vi "myRIO_BRig_Host_v0,30.vi"() -> ()   [LabVIEW 2014]
panel:
  out "element":u16
  out "error_LoadPrevSettings":errorcluster caption="error out"
  in  "LoadPrevSettings":bool
  out "RunTime_seconds":u16
  out "RunTime_minutes":u16
  out "BlockL_T2R_cur":u16 caption="Trials2Reward"
  out "BlockL_BTPR_cur":u16 caption="BadTrialsPostReward"
  out "BlockL_T2R_avg":dbl caption="Trials2Reward" format="%#_3g"
  out "BlockL_BTPR_avg":dbl caption="BadTrialsPostReward" format="%#_3g"
  out "BlockR_T2R_cur":u16 caption="Trials2Reward"
  out "BlockR_BTPR_cur":u16 caption="BadTrialsPostReward"
  out "BlockR_T2R_avg":dbl caption="Trials2Reward" format="%#_3g"
  out "BlockR_BTPR_avg":dbl caption="BadTrialsPostReward" format="%#_3g"
  out "graph_ai1":dbl(graph)
  out "graph_ai0":dbl(graph)
  in  "dataIn_maxTrialsDisplayed":i32 caption="Number of Trials Displayed\n( 0 = all trials )"
  out "error_TCP":errorcluster
  in  "stop":bool
  in  "colorIn_timeout":u32(colorbox)=7468543 caption="Choice Timeout"
  in  "colorIn_wrong/cue":u32(colorbox)=16728618 caption="Wrong Choice or\nLicked During Cue"
  in  "colorIn_reward":u32(colorbox)=5898088 caption="Reward"
  in  "colorIn_unknown":u32(colorbox)=16449331 caption="Unknown Trial Status"
  out "dataOut_plot":cluster{i32[], i32[]}[](graph)
  out "iTrial":i32
  out "iBlock":i32
  # "Exp Stats"
  # "Current Block Stats"
  # "Trials 2 Reward\n\nBad Trials\nPost Reward"
  # "Left Spout    Right Spout"
  # "Run Time\n\n   minutes    seconds"
  # "Average Block Stats"
  # "Trials 2 Reward\n\nBad Trials\nPost Reward"
  # "Left Spout    Right Spout"
  # "If you get ERROR 5 related to opening a file, press CONTINUE"
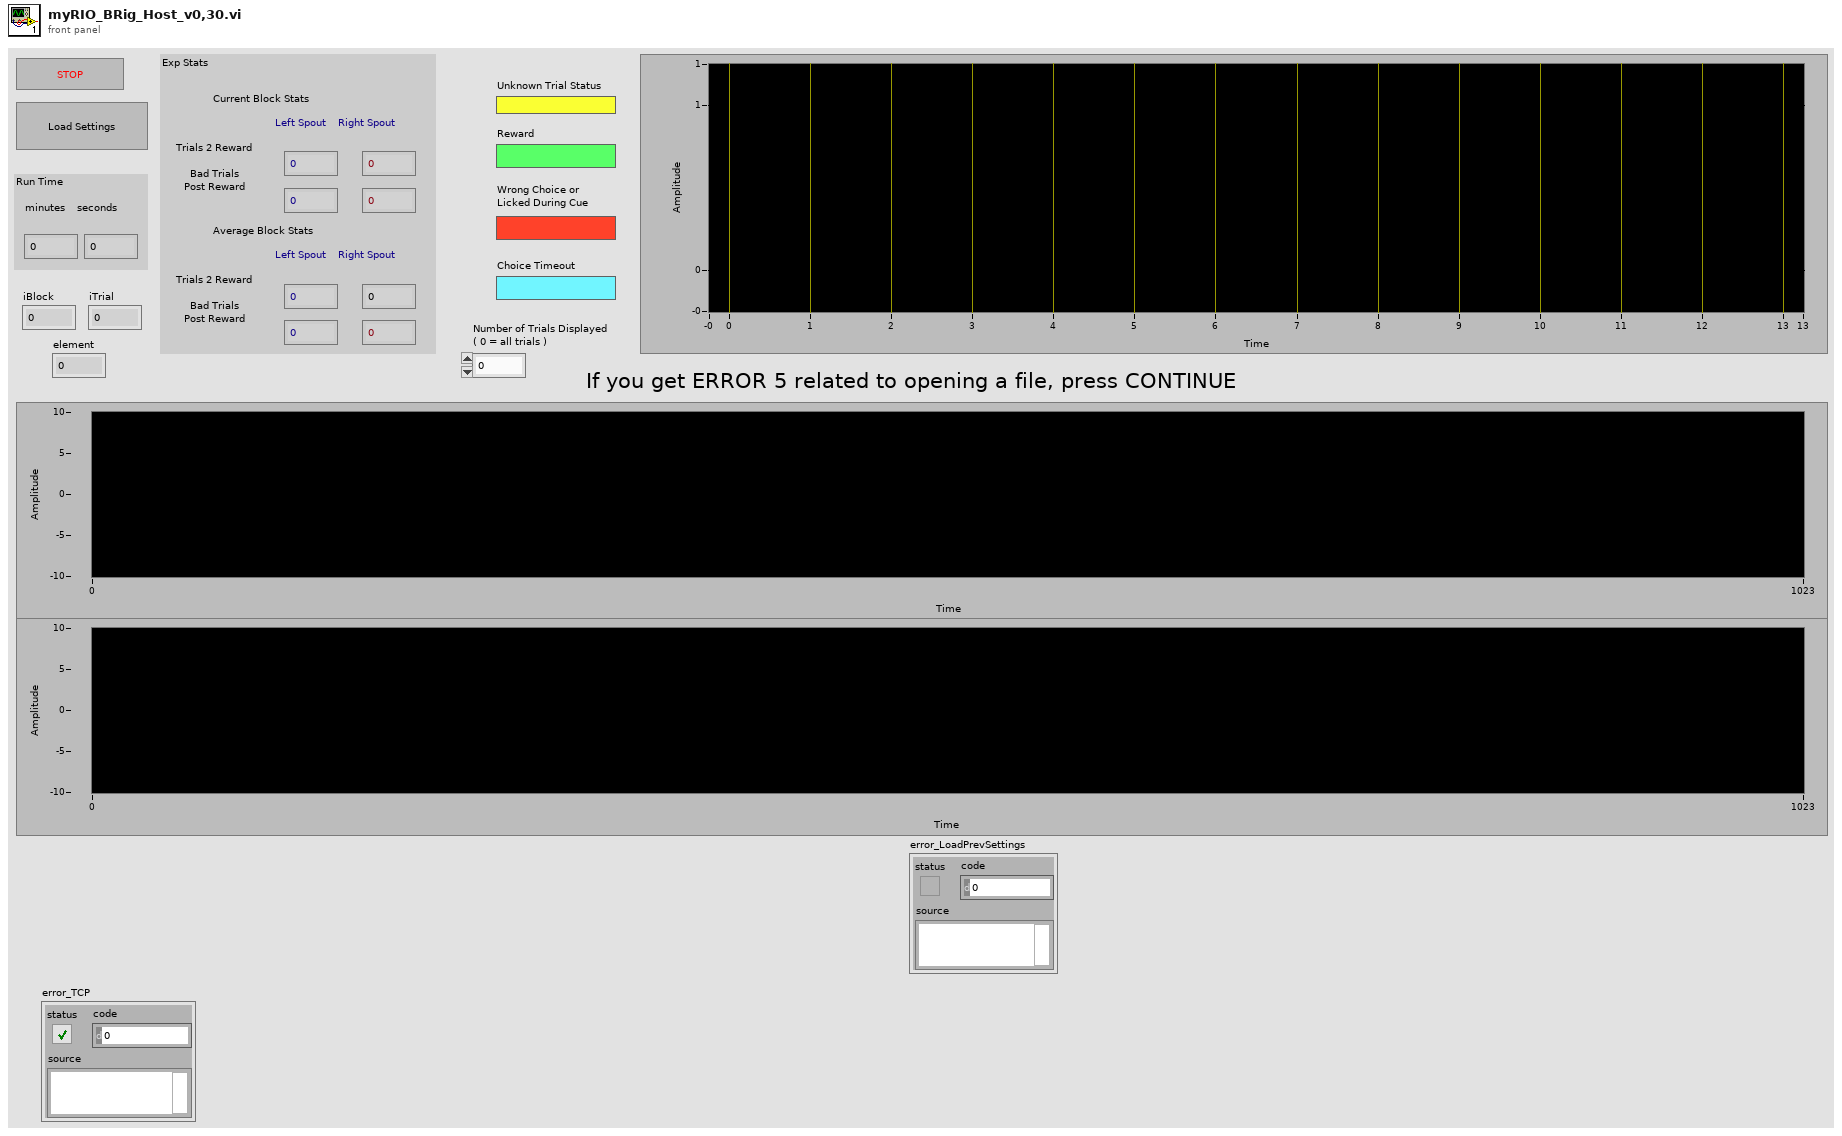
[diagram p1: front panel]
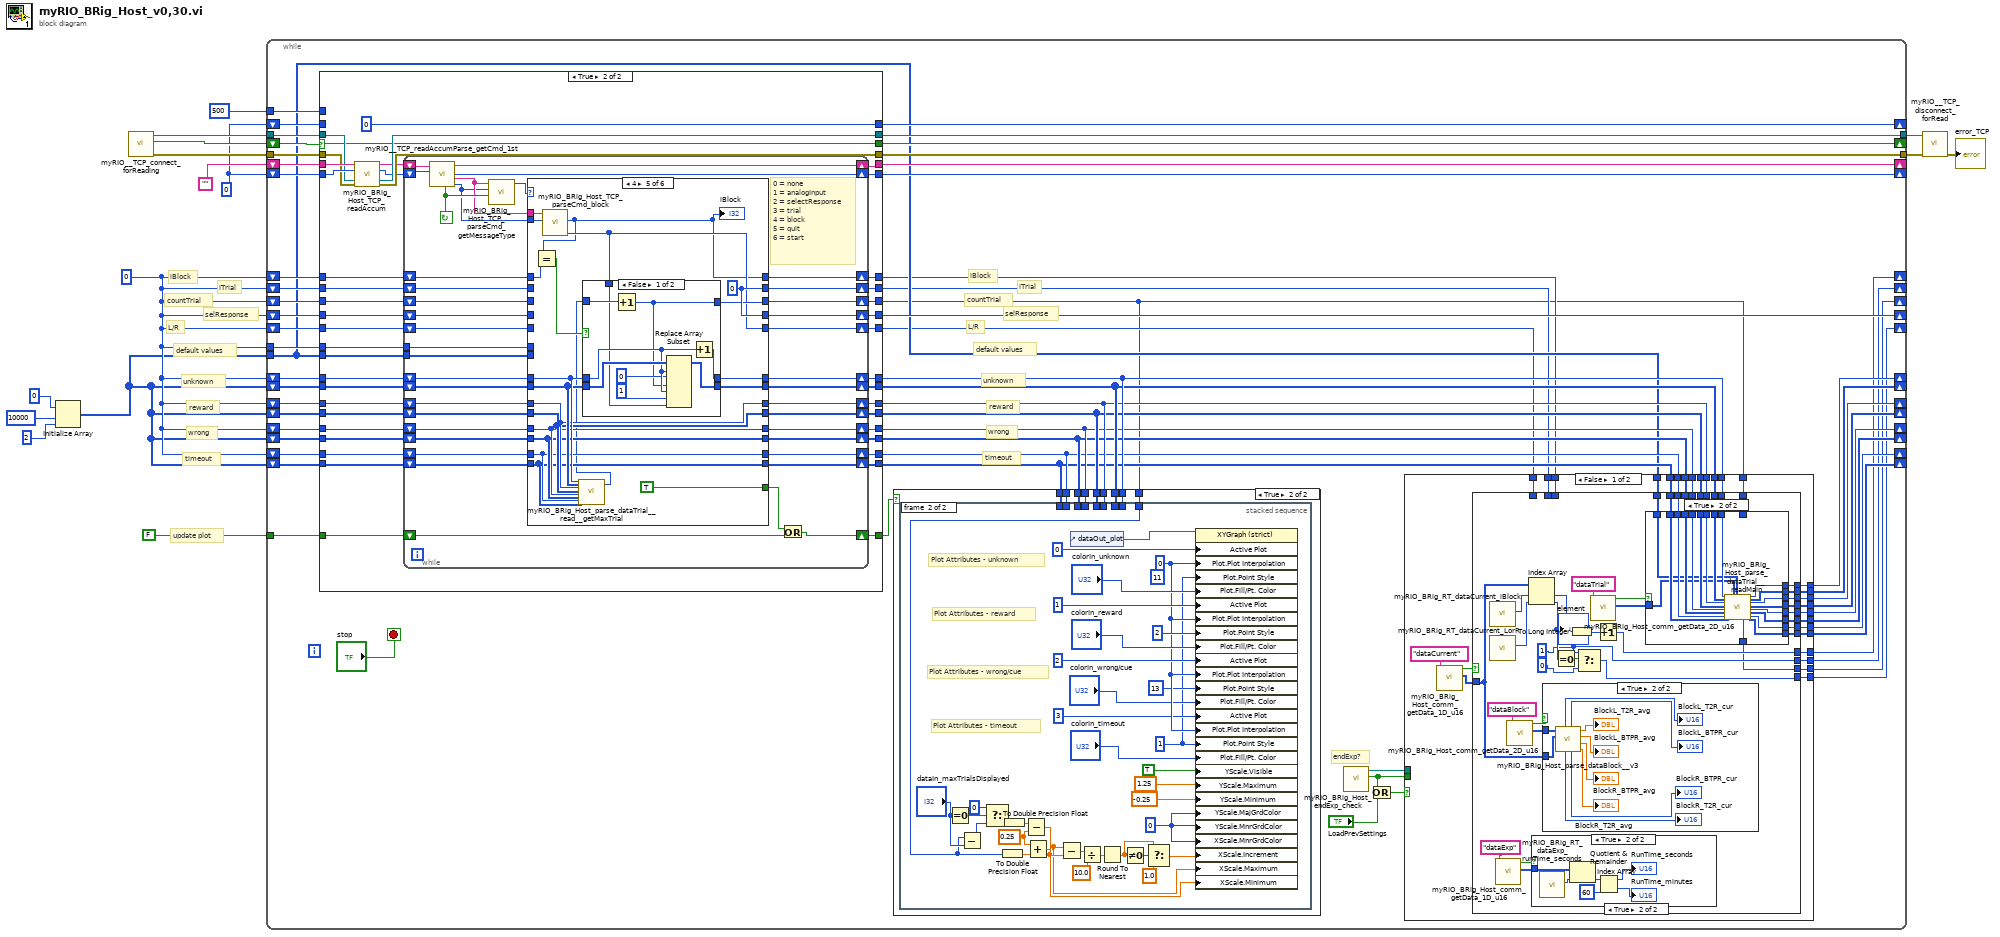
[diagram p0: block diagram]
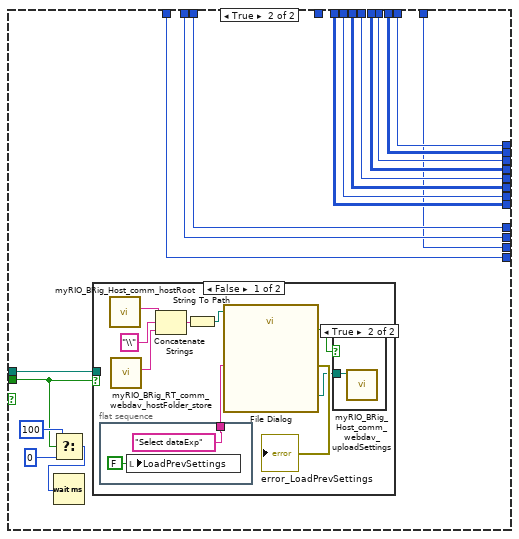
[diagram p6: hidden frame]
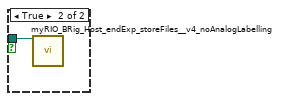
[diagram p8: hidden frame]
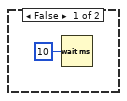
[diagram p9: hidden frame]
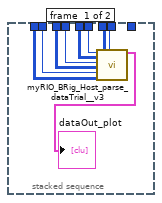
[diagram p10: hidden frame]
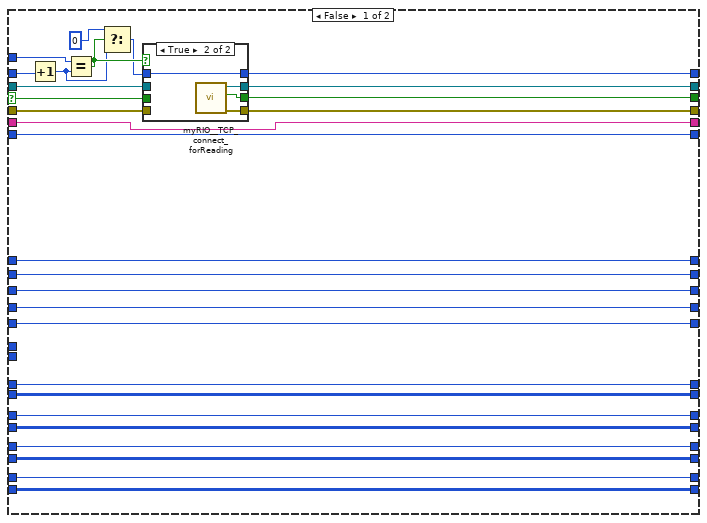
[diagram p11: hidden frame]
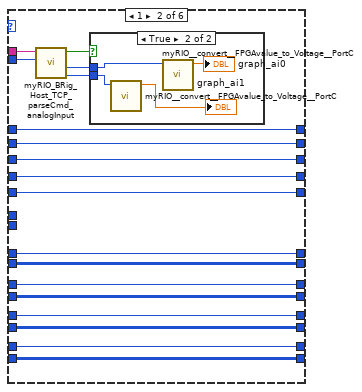
[diagram p14: hidden frame]
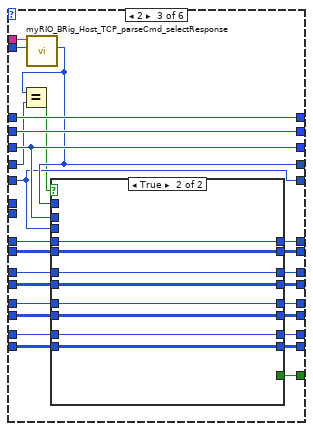
[diagram p16: hidden frame]
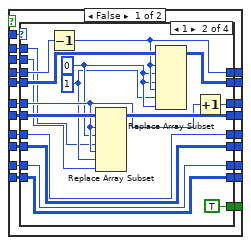
[diagram p17: hidden frame]
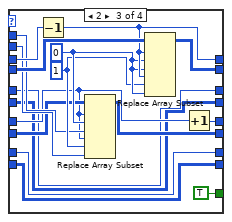
[diagram p19: hidden frame]
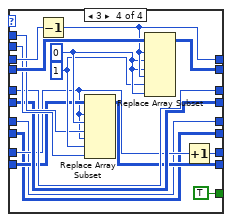
[diagram p20: hidden frame]
diagram:
  w2 = 0
  w11 = 0
  # "default values"
  # "update plot"
  # "timeout"
  # "wrong"
  # "reward"
  # "unknown"
  # "L/R"
  # "selResponse"
  # "countTrial"
  # "iBlock"
  # "iTrial"
  n1 = Initialize Array(0 ("element"), 10000 ("dimension size"), 2 ("dimension size")) -> (w1:i32[][])
  n2 = call "myRIO__TCP_connect_forReading.vi"() -> ("output_error"=w13:errorcluster, "output_connected"=w14:bool, "output_hTCP"=w15:refnum<k5>)  [unwired: 9 in]
  n3 = while {
    tunnel: w15 -> [w74]
    tunnel: w13 -> [w72]
    shift-right: [w65] -> _
    shift-left: w11 -> [w70]
    shift-right: [w66] -> _
    shift-left: "" -> [w71]
    shift-right: [w67] -> _
    shift-left: w14 -> [w73]
    shift-right: [w68] -> _
    shift-left: w11 -> [w75]
    tunnel: 500 ("y") -> [w69]
    shift-right: [w18] -> _
    shift-left: w2 -> [w64]
    shift-right: [w19] -> _
    shift-left: w2 -> [w63]
    shift-right: [w16] -> _
    shift-left: w2 -> [w62]
    shift-right: [w50] -> _
    shift-left: w2 -> [w61]
    shift-right: [w23] -> _
    shift-left: w2 -> [w60]
    shift-right: [w31] -> _
    shift-left: w2 -> [w59]
    shift-right: [w30] -> _
    shift-left: w1 -> [w58]
    shift-right: [w29] -> _
    shift-left: w2 -> [w57]
    shift-right: [w28] -> _
    shift-left: w1 -> [w56]
    shift-right: [w27] -> _
    shift-left: w2 -> [w55]
    shift-right: [w26] -> _
    shift-left: w1 -> [w54]
    shift-right: [w25] -> _
    shift-left: w2 -> [w53]
    shift-right: [w24] -> _
    shift-left: w1 -> [w52]
    tunnel: [w48] -> w5
    tunnel: [w47] -> w4
    tunnel: FALSE -> [w51]
    tunnel: w2 -> [w45]
    tunnel: w1 -> [w32]
    stop <- "stop" stop-if-true
    # "default values"
    # "timeout"
    # "wrong"
    # "reward"
    # "unknown"
    # "L/R"
    # "selResponse"
    # "countTrial"
    # "iBlock"
    # "iTrial"
    # "endExp?"
    n4 = case shown="True" w73 {
      selector: w73 -> [w305 w354]
      tunnel: w71 -> [w299 w360]
      tunnel: w70 -> [w300 w359]
      tunnel: [w299 w350] -> w66
      tunnel: [w300 w349] -> w65
      tunnel: w74 -> [w306 w358]
      tunnel: [w309 w357] -> w48
      tunnel: w72 -> [w304 w356]
      tunnel: [w308 w355] -> w47
      tunnel: [w307 w354] -> w67
      tunnel: w75 -> [w310 _]
      tunnel: [w298 0] -> w68
      tunnel: w69 -> [w297 _]
      tunnel: w64 -> [w296 w348]
      tunnel: w63 -> [w295 w347]
      tunnel: w62 -> [w294 w346]
      tunnel: w61 -> [w293 w345]
      tunnel: w60 -> [w292 w344]
      tunnel: w59 -> [w291 w343]
      tunnel: w58 -> [w290 w342]
      tunnel: w57 -> [w289 w341]
      tunnel: w56 -> [w288 w340]
      tunnel: w55 -> [w287 w339]
      tunnel: w54 -> [w286 w338]
      tunnel: w53 -> [w285 w337]
      tunnel: w52 -> [w284 w336]
      tunnel: w51 -> [_ w335]
      tunnel: [_ w334] -> w49
      tunnel: [w296 w333] -> w22
      tunnel: [w295 w332] -> w21
      tunnel: [w294 w331] -> w17
      tunnel: [w293 w330] -> w50
      tunnel: [w292 w329] -> w20
      tunnel: [w291 w328] -> w40
      tunnel: [w290 w327] -> w39
      tunnel: [w289 w326] -> w38
      tunnel: [w288 w325] -> w37
      tunnel: [w287 w324] -> w36
      tunnel: [w286 w323] -> w35
      tunnel: [w285 w322] -> w34
      tunnel: [w284 w321] -> w33
      tunnel: w45 -> [_ w320]
      tunnel: w32 -> [_ w319]
      frame False {
        n5 = Increment(x=w310) -> (x+1=w283:i32)
        n6 = Equal?(x=w297, y=w283) -> (x = y?=w303:bool)
        n7 = Select(t=0, s=w303, f=w283) -> (s? t:f=w301:i32)
        n8 = case shown="True" w303 {
          tunnel: w301 -> [w311 w315]
          tunnel: [w314 w318] -> w309
          tunnel: [w312 w317] -> w308
          tunnel: [w313 w316] -> w307
          tunnel: w306 -> [w314 _]
          tunnel: w305 -> [w313 _]
          tunnel: w304 -> [w312 _]
          tunnel: [w311 w315] -> w298
          frame False {
          }
          frame True {
            n9 = call "myRIO__TCP_connect_forReading.vi"() -> ("output_error"=w317:errorcluster, "output_connected"=w316:bool, "output_hTCP"=w318:refnum<k5>)  [unwired: 9 in]
          }
        }
      }
      frame True {
        n10 = call "myRIO_BRig_Host_TCP_readAccum.vi"("input_strAccum"=w360, "input_count"=w359, "input_handle_TCP"=w358, "input_error"=w356) -> ("output_strAccum"=w352:string, "output_count"=w351:i32, "output_handle_TCP"=w357:refnum<k5>, "output_error"=w355:errorcluster)  [unwired: 8 in]
        n11 = while {
          shift-right: [w397] -> w350
          shift-left: w352 -> [w399]
          shift-right: [w396] -> w349
          shift-left: w351 -> [w398]
          shift-right: [w388] -> w333
          shift-left: w348 -> [w391]
          shift-right: [w387] -> w332
          shift-left: w347 -> [w390]
          shift-right: [w386] -> w331
          shift-left: w346 -> [w389]
          shift-right: [w384] -> w330
          shift-left: w345 -> [w385]
          shift-right: [w382] -> w329
          shift-left: w344 -> [w383]
          shift-right: [w380] -> w328
          shift-left: w343 -> [w381]
          shift-right: [w378] -> w327
          shift-left: w342 -> [w379]
          shift-right: [w371] -> w326
          shift-left: w341 -> [w377]
          shift-right: [w370] -> w325
          shift-left: w340 -> [w376]
          shift-right: [w369] -> w324
          shift-left: w339 -> [w375]
          shift-right: [w368] -> w323
          shift-left: w338 -> [w374]
          shift-right: [w366] -> w321
          shift-left: w336 -> [w372]
          shift-right: [w367] -> w322
          shift-left: w337 -> [w373]
          shift-right: [w363] -> w334
          shift-left: w335 -> [w365]
          tunnel: w320 -> [w362]
          tunnel: w319 -> [w361]
          stop <- w395 continue-if-true
          # "0 = none\n1 = analogInput\n2 = selectResponse\n3 = trial\n4 = block\n5 = quit\n6 = start"
          n12 = call "myRIO__TCP_readAccumParse_getCmd_1st.vi"("input_count"=w398, "input_strAccum"=w399) -> ("output_countCmd"=w393:i32, "output_strCmd"=w394:string, "output_count"=w396:i32, "output_strAccum"=w397:string, "output_haveCmd"=w395:bool)  [unwired: 5 in]
          n13 = call "myRIO_BRig_Host_TCP_parseCmd_getMessageType.vi"("input_haveCmd"=w395, "input_countCmd"=w393, "input_strCmd"=w394) -> ("output_messageType"=w392:u8)  [unwired: 8 in]
          n14 = case shown="4" w392 {
            tunnel: w394 -> [_ w417 w459 w570 w602 w649]
            tunnel: w393 -> [_ w416 w458 w569 w601 _]
            tunnel: w391 -> [w412 w430 w460 w567 w595 w644]
            tunnel: w390 -> [w411 w429 w441 w561 _ w642]
            tunnel: w389 -> [w410 w428 w440 _ _ w641]
            tunnel: [w412 w430 w460 w567 w593 w643] -> w388
            tunnel: [w411 w429 w441 w560 w603 w638] -> w387
            tunnel: [w410 w428 w440 w564 w597 w637] -> w386
            tunnel: w385 -> [w409 w427 w438 _ _ w640]
            tunnel: [w409 w427 w437 0 ("output_iTrial_num") w603 w636] -> w384
            tunnel: w383 -> [w408 w426 w436 w563 _ w639]
            tunnel: [w408 w426 w436 w563 w596 w635] -> w382
            tunnel: w381 -> [w407 w425 w456 w549 w592 w634]
            tunnel: [w407 w425 w454 w566 w599 w626] -> w380
            tunnel: w379 -> [w406 w424 w457 w550 w591 w633]
            tunnel: [w406 w424 w455 w565 w600 w625] -> w378
            tunnel: w377 -> [w405 w423 w453 w551 w590 w632]
            tunnel: w376 -> [w404 w422 w452 w552 w589 w631]
            tunnel: w375 -> [w403 w421 w451 w553 w588 w630]
            tunnel: w374 -> [w402 w420 w450 w554 w587 w629]
            tunnel: w373 -> [w401 w419 w449 w555 w586 w628]
            tunnel: w372 -> [w400 w418 w448 w556 w585 w627]
            tunnel: [w405 w423 w442 w551 w590 w624] -> w371
            tunnel: [w404 w422 w443 w552 w589 w623] -> w370
            tunnel: [w403 w421 w444 w553 w588 w622] -> w369
            tunnel: [w402 w420 w445 w554 w587 w621] -> w368
            tunnel: [w401 w419 w446 w555 w586 w620] -> w367
            tunnel: [w400 w418 w447 w556 w585 w619] -> w366
            tunnel: [_ _ w439 w562 TRUE w616] -> w364
            tunnel: w362 -> [_ _ _ _ _ w618]
            tunnel: w361 -> [_ _ _ _ _ w617]
            frame 0, Default {
            }
            frame 1 {
              n15 = call "myRIO_BRig_Host_TCP_parseCmd_analogInput.vi"("input_countCmd"=w416, "input_strCmd"=w417) -> ("output_ai1"=w413:i32, "output_ai0"=w414:i32, "output_haveAnalogInput"=w415:bool)  [unwired: 7 in]
              n16 = case shown="True" w415 {
                tunnel: w414 -> [_ w434]
                tunnel: w413 -> [_ w432]
                frame False {
                }
                frame True {
                  n17 = call "myRIO__convert__FPGAvalue_to_Voltage__PortC.vi"("input_FPGAvalue_PortC"=w432) -> ("output_voltage"=→"graph_ai1":dbl)  [unwired: 10 in]
                  n18 = call "myRIO__convert__FPGAvalue_to_Voltage__PortC.vi"("input_FPGAvalue_PortC"=w434) -> ("output_voltage"=→"graph_ai0":dbl)  [unwired: 10 in]
                }
              }
            }
            frame 2 {
              n19 = call "myRIO_BRig_Host_TCP_parseCmd_selectResponse.vi"("input_countCmd"=w458, "input_strCmd"=w459) -> ("output_selectResponse_num"=w437:i32)  [unwired: 8 in, 1 out]
              n20 = Equal?(x=w437, y=w438) -> (x = y?=w435:bool)
              n21 = case shown="True" w435 {
                tunnel: w457 -> [w480 w546]
                tunnel: w456 -> [w479 w547]
                tunnel: [w478 w546] -> w455
                tunnel: [w477 w547] -> w454
                tunnel: w453 -> [w476 w545]
                tunnel: w452 -> [w475 w544]
                tunnel: w451 -> [w474 w543]
                tunnel: w450 -> [w473 w542]
                tunnel: w449 -> [w472 w541]
                tunnel: w448 -> [w471 w540]
                tunnel: [w470 w540] -> w447
                tunnel: [w469 w541] -> w446
                tunnel: [w468 w542] -> w445
                tunnel: [w467 w543] -> w444
                tunnel: [w466 w544] -> w443
                tunnel: [w465 w545] -> w442
                tunnel: w440 -> [w464 _]
                tunnel: [w463 _] -> w439
                tunnel: w437 -> [w462 _]
                tunnel: w436 -> [w461 _]
                frame False {
                  n22 = case shown="1" w462 {
                    tunnel: w480 -> [w487 w500 w520 w537]
                    tunnel: w479 -> [w488 w505 w522 w539]
                    tunnel: [w487 w499 w519 w536] -> w478
                    tunnel: [w488 w498 w518 w535] -> w477
                    tunnel: w476 -> [w481 w493 w506 w529]
                    tunnel: w475 -> [w482 w495 w507 w530]
                    tunnel: w474 -> [w483 w502 w510 w523]
                    tunnel: w473 -> [w484 w503 w511 w524]
                    tunnel: w472 -> [w485 w496 w516 w527]
                    tunnel: w471 -> [w486 w497 w517 w528]
                    tunnel: [w486 w497 w517 w525] -> w470
                    tunnel: [w485 w496 w516 w526] -> w469
                    tunnel: [w484 w503 w508 w524] -> w468
                    tunnel: [w483 w502 w509 w523] -> w467
                    tunnel: [w482 w494 w507 w530] -> w466
                    tunnel: [w481 w504 w506 w529] -> w465
                    tunnel: w464 -> [_ w490 w513 w532]
                    tunnel: [_ TRUE TRUE TRUE] -> w463
                    tunnel: w461 -> [_ w489 w512 w531]
                    frame 0, Default {
                    }
                    frame 1 {
                      w491 = 1 ("new element/subarray")
                      w492 = 0 ("new element/subarray")
                      n23 = Decrement(x=w505) -> (x-1=w498:i32)
                      n24 = Replace Array Subset(array=w495, new element #1=w490, index (row) #1=w493, index (col) #1=w492, new element #2=w489, index (row) #2=w493, index (col) #2=w491) -> (w494:i32[][])
                      n25 = Replace Array Subset(array=w500, new element #1=w492, index (row) #1=w498, index (col) #1=w492, new element #2=w492, index (row) #2=w498, index (col) #2=w491) -> (w499:i32[][])
                      n26 = Increment(x=w493) -> (x+1=w504:i32)
                    }
                    frame 2 {
                      w514 = 1 ("new element/subarray")
                      w515 = 0 ("new element/subarray")
                      n27 = Decrement(x=w522) -> (x-1=w518:i32)
                      n28 = Replace Array Subset(array=w511, new element #1=w513, index (row) #1=w510, index (col) #1=w515, new element #2=w512, index (row) #2=w510, index (col) #2=w514) -> (w508:i32[][])
                      n29 = Replace Array Subset(array=w520, new element #1=w515, index (row) #1=w518, index (col) #1=w515, new element #2=w515, index (row) #2=w518, index (col) #2=w514) -> (w519:i32[][])
                      n30 = Increment(x=w510) -> (x+1=w509:i32)
                    }
                    frame 3 {
                      w533 = 1 ("new element/subarray")
                      w534 = 0 ("new element/subarray")
                      n31 = Decrement(x=w539) -> (x-1=w535:i32)
                      n32 = Replace Array Subset(array=w528, new element #1=w532, index (row) #1=w527, index (col) #1=w534, new element #2=w531, index (row) #2=w527, index (col) #2=w533) -> (w525:i32[][])
                      n33 = Replace Array Subset(array=w537, new element #1=w534, index (row) #1=w535, index (col) #1=w534, new element #2=w534, index (row) #2=w535, index (col) #2=w533) -> (w536:i32[][])
                      n34 = Increment(x=w527) -> (x+1=w526:i32)
                    }
                  }
                }
                frame True {
                }
              }
            }
            frame 3 {
              n35 = Equal To 0?(x=w561) -> (x = 0?=w558:bool)
              n36 = call "myRIO_BRig_Host_TCP_parseCmd_trial.vi"("input_countCmd"=w569, "input_strCmd"=w570) -> ("output_iTrial_num"=w560:i32)  [unwired: 8 in, 1 out]
              "iTrial" <- w560
              n37 = Equal?(x=w560, y=w561) -> (x = y?=w559:bool)
              n38 = Or(x=w559, y=w558) -> (x .or. y?=w557:bool)
              n39 = call "myRIO_BRig_Host_parse_dataTrial__read__getMaxTrial.vi"("input_idxUnknown"=w549, "input_arrayUnknown"=w550, "input_idxReward"=w551, "input_arrayReward"=w552, "input_idxWrong"=w553, "input_arrayWrong"=w554, "input_idxTimeout"=w555, "input_arrayTimeout"=w556) -> ("output_maxTrial"=w548:i32)  [unwired: 19 in]
              n40 = case shown="False" w557 {
                tunnel: w549 -> [w579 w583]
                tunnel: w550 -> [w580 w582]
                tunnel: w548 -> [w574 w581]
                tunnel: [w578 w583] -> w566
                tunnel: [w577 w582] -> w565
                tunnel: [w573 w581] -> w564
                tunnel: w563 -> [w572 _]
                tunnel: [TRUE _] -> w562
                frame False {
                  n41 = Increment(x=w574) -> (x+1=w573:i32)
                  n42 = Replace Array Subset(array=w580, new element #1=w573, index (row) #1=w579, index (col) #1=0 ("new element/subarray"), new element #2=w572, index (row) #2=w579, index (col) #2=1 ("new element/subarray")) -> (w577:i32[][])
                  n43 = Increment(x=w579) -> (x+1=w578:i32)
                }
                frame True {
                }
              }
            }
            frame 4 {
              w603 = 0 ("output_iTrial_num")
              n44 = call "myRIO_BRig_Host_TCP_parseCmd_block.vi"("input_countCmd"=w601, "input_strCmd"=w602) -> ("output_L_or_R"=w596:i32, "output_iBlock_num"=w593:i32)  [unwired: 7 in, 1 out]
              "iBlock" <- w593
              n45 = Equal?(x=w593, y=w595) -> (x = y?=w594:bool)
              n46 = call "myRIO_BRig_Host_parse_dataTrial__read__getMaxTrial.vi"("input_idxUnknown"=w592, "input_arrayUnknown"=w591, "input_idxReward"=w590, "input_arrayReward"=w589, "input_idxWrong"=w588, "input_arrayWrong"=w587, "input_idxTimeout"=w586, "input_arrayTimeout"=w585) -> ("output_maxTrial"=w584:i32)  [unwired: 19 in]
              n47 = case shown="False" w594 {
                tunnel: w584 -> [w612 w613]
                tunnel: w591 -> [w611 w614]
                tunnel: [w610 w614] -> w600
                tunnel: [w609 w615] -> w599
                tunnel: w592 -> [w608 w615]
                tunnel: w596 -> [w605 _]
                tunnel: [w604 w613] -> w597
                frame False {
                  n48 = Increment(x=w612) -> (x+1=w604:i32)
                  n49 = Replace Array Subset(array=w611, new element #1=w604, index (row) #1=w608, index (col) #1=0 ("new element/subarray"), new element #2=w605, index (row) #2=w608, index (col) #2=1 ("new element/subarray")) -> (w610:i32[][])
                  n50 = Increment(x=w608) -> (x+1=w609:i32)
                }
                frame True {
                }
              }
            }
            frame 6 {
              n51 = String Subset(string=w649, offset (0)=2, length (rest)=1 ("length (rest)")) -> (substring=w646:string)
              n52 = Equal?(x=w646, y="e") -> (x = y?=w616:bool)
              n53 = case shown="True" w616 {
                tunnel: w644 -> [w662 _]
                tunnel: [w662 w664] -> w643
                tunnel: w642 -> [w661 _]
                tunnel: w641 -> [w660 _]
                tunnel: w640 -> [w659 _]
                tunnel: w639 -> [w658 _]
                tunnel: [w661 w664] -> w638
                tunnel: [w660 w664] -> w637
                tunnel: [w659 w664] -> w636
                tunnel: [w658 w664] -> w635
                tunnel: w634 -> [w657 _]
                tunnel: w633 -> [w656 _]
                tunnel: w632 -> [w655 _]
                tunnel: w631 -> [w654 _]
                tunnel: w630 -> [w653 _]
                tunnel: w629 -> [w652 _]
                tunnel: w628 -> [w651 _]
                tunnel: w627 -> [w650 _]
                tunnel: [w657 w664] -> w626
                tunnel: [w656 w663] -> w625
                tunnel: [w655 w664] -> w624
                tunnel: [w654 w663] -> w623
                tunnel: [w653 w664] -> w622
                tunnel: [w652 w663] -> w621
                tunnel: [w651 w664] -> w620
                tunnel: [w650 w663] -> w619
                tunnel: w618 -> [_ w664]
                tunnel: w617 -> [_ w663]
                frame False {
                }
                frame True {
                }
              }
            }
          }
          n54 = Or(x=w364, y=w365) -> (x .or. y?=w363:bool)
        }
      }
    }
    n55 = case shown="True" w49 {
      tunnel: w33 -> [_ w238]
      tunnel: w34 -> [_ w237]
      tunnel: w35 -> [_ w236]
      tunnel: w36 -> [_ w235]
      tunnel: w37 -> [_ w234]
      tunnel: w38 -> [_ w233]
      tunnel: w39 -> [_ w232]
      tunnel: w40 -> [_ w231]
      tunnel: w17 -> [_ w230]
      frame False {
        n56 = Wait (ms)(milliseconds to wait=u32 10) -> ()  [unwired: 1 out]
      }
      frame True {
        n57 = stacked-sequence {
          tunnel: w238 -> [w247 _]
          tunnel: w237 -> [w246 _]
          tunnel: w236 -> [w245 _]
          tunnel: w235 -> [w244 _]
          tunnel: w234 -> [w243 _]
          tunnel: w233 -> [w242 _]
          tunnel: w232 -> [w241 _]
          tunnel: w231 -> [w240 _]
          tunnel: w230 -> [_ w256]
          frame #0 {
            n58 = call "myRIO_BRig_Host_parse_dataTrial__v3.vi"("input_idxReward"=w242, "input_arrayReward"=w243, "input_idxWrong"=w244, "input_arrayWrong"=w245, "input_idxTimeout"=w246, "input_arrayTimeout"=w247, "input_arrayUnknown"=w241, "input_idxUnknown"=w240) -> ("output_plotData"=→"dataOut_plot":cluster{i32[], i32[]}[])  [unwired: 11 in]
          }
          frame #1 {
            w252 = u32 0 ("Y Scale.Grid Colors:Major Color")
            w260 = 0.25 ("y")
            w249 = u8 1 ("Plot.Point Style")
            (unwired) u8 11 ("Plot.Point Style")
            w276 = u8 0 ("Plot.Plot Interpolation")
            # "Plot Attributes - timeout"
            # "Plot Attributes - wrong/cue"
            # "Plot Attributes - reward"
            # "Plot Attributes - unknown"
            n59 = Equal To 0?(x="dataIn_maxTrialsDisplayed") -> (x = 0?=w257:bool)
            n60 = Subtract(x=w256, y="dataIn_maxTrialsDisplayed") -> (x-y=w258:i32)
            n61 = Select(t=0, s=w257, f=w258) -> (s? t:f=w263:i32)
            n62 = To Double Precision Float(number=w256) -> (double precision float=w261:dbl)
            n63 = To Double Precision Float(number=w263) -> (double precision float=w262:dbl)
            n64 = Subtract(x=w262, y=w260) -> (x-y=w250:dbl)
            n65 = Add(x=w260, y=w261) -> (x+y=w248:dbl)
            n66 = Subtract(x=w248, y=w250) -> (x-y=w264:dbl)
            n67 = control-ref of="dataOut_plot"() -> (w271:refnum<vi>)
            n68 = Divide(x=w264, y=10.0) -> (x/y=w266:dbl)
            n69 = Round To Nearest(number=w266) -> (nearest integer value=w268:dbl)
            n70 = Not Equal To 0?(x=w268) -> (x != 0?=w267:bool)
            n71 = Select(t=w268, s=w267, f=1.0) -> (s? t:f=w251:dbl)
            n72 = property on="Property Node" class="XYGraph (strict)"(reference=w271, "Active Plot"=u32 0, "Plot.Plot Interpolation"=w276, "Plot.Point Style"=w249, "Plot.Fill/Pt. Color"="colorIn_unknown", "Active Plot"=u32 1, "Plot.Plot Interpolation"=w276, "Plot.Point Style"=u8 2, "Plot.Fill/Pt. Color"="colorIn_reward", "Active Plot"=u32 2, "Plot.Plot Interpolation"=w276, "Plot.Point Style"=u8 13, "Plot.Fill/Pt. Color"="colorIn_wrong/cue", "Active Plot"=u32 3, "Plot.Plot Interpolation"=w276, "Plot.Point Style"=w249, "Plot.Fill/Pt. Color"="colorIn_timeout", "YScale.Visible"=TRUE ("Y Scale.Visible"), "YScale.Maximum"=1.25 ("Y Scale.Range:Maximum"), "YScale.Minimum"=-0.25 ("Y Scale.Range:Minimum"), "YScale.MajGrdColor"=w252, "YScale.MnrGrdColor"=w252, "XScale.MnrGrdColor"=w252, "XScale.Increment"=w251, "XScale.Maximum"=w248, "XScale.Minimum"=w250) -> ()  [unwired: 1 in, 2 out]
          }
        }
      }
    }
    n73 = call "myRIO_BRig_Host_endExp_check.vi"() -> ("output_IendExp"=w42:bool, "output_filePath_expExp"=w41:path)  [unwired: 10 in]
    n74 = Or(x=w42, y="LoadPrevSettings") -> (x .or. y?=w43:bool)
    n75 = case shown="False" w43 {
      tunnel: w42 -> [_ w212]
      tunnel: w41 -> [_ w211]
      tunnel: [w100 w210] -> w31
      tunnel: [w99 w209] -> w30
      tunnel: [w98 w208] -> w29
      tunnel: [w97 w207] -> w28
      tunnel: [w96 w206] -> w27
      tunnel: [w95 w205] -> w26
      tunnel: [w94 w204] -> w25
      tunnel: [w93 w203] -> w24
      tunnel: w40 -> [w92 w210]
      tunnel: w39 -> [w91 w209]
      tunnel: w38 -> [w90 w208]
      tunnel: w37 -> [w89 w207]
      tunnel: w36 -> [w88 w206]
      tunnel: w35 -> [w87 w205]
      tunnel: w34 -> [w86 w204]
      tunnel: w33 -> [w85 w203]
      tunnel: w32 -> [w84 _]
      tunnel: [w83 w200] -> w23
      tunnel: [w82 w201] -> w19
      tunnel: [w81 w202] -> w18
      tunnel: w22 -> [w80 w202]
      tunnel: w21 -> [w79 w201]
      tunnel: w20 -> [w78 w200]
      tunnel: [w77 w199] -> w16
      tunnel: w17 -> [w76 w199]
      frame False {
        n76 = call "myRIO_BRig_Host_comm_getData_1D_u16.vi"("input_fileName"="dataCurrent") -> ("output_data_1D"=w101:u16[], "output_I_data"=w102:bool)  [unwired: 9 in]
        n77 = case shown="True" w102 {
          tunnel: w101 -> [_ w151]
          tunnel: [w115 w143] -> w100
          tunnel: [w114 w142] -> w99
          tunnel: [w113 w141] -> w98
          tunnel: [w112 w140] -> w97
          tunnel: [w111 w139] -> w96
          tunnel: [w110 w138] -> w95
          tunnel: [w109 w137] -> w94
          tunnel: [w108 w136] -> w93
          tunnel: w92 -> [w115 w135]
          tunnel: w91 -> [w114 w134]
          tunnel: w90 -> [w113 w133]
          tunnel: w89 -> [w112 w132]
          tunnel: w88 -> [w111 w131]
          tunnel: w87 -> [w110 w130]
          tunnel: w86 -> [w109 w129]
          tunnel: w85 -> [w108 w128]
          tunnel: w84 -> [_ w127]
          tunnel: [w105 w123] -> w83
          tunnel: [w106 w122] -> w82
          tunnel: [w107 w118] -> w81
          tunnel: w80 -> [w107 _]
          tunnel: w79 -> [w106 _]
          tunnel: w78 -> [w105 _]
          tunnel: [w104 w117] -> w77
          tunnel: w76 -> [w104 w116]
          frame False {
          }
          frame True {
            w122 = 1
            n78 = call "myRIO_BRig_RT_dataCurrent_iBlock.vi"() -> ("output_iBlock"=w121:i32)  [unwired: 11 in]
            n79 = call "myRIO_BRig_RT_dataCurrent_LorR.vi"() -> ("output_LorR"=w144:i32)  [unwired: 11 in]
            n80 = call "myRIO_BRig_Host_comm_getData_1D_u16.vi"("input_fileName"="dataExp") -> ("output_data_1D"=w148:u16[], "output_I_data"=w149:bool)  [unwired: 9 in]
            n81 = call "myRIO_BRig_Host_comm_getData_2D_u16.vi"("input_fileName"="dataBlock") -> ("output_data_2D"=w152:u16[][], "output_I_data"=w153:bool)  [unwired: 9 in]
            n82 = Index Array(array=w151, index #1=w121, index #2=w144) -> (element #1=w120:u16, element #2=w126:u16)
            "element" <- w126
            n83 = case shown="True" w149 {
              tunnel: w148 -> [_ w188]
              frame False {
              }
              frame True {
                n84 = call "myRIO_BRig_RT_dataExp_runTime_seconds.vi"() -> ("output_RunTime_minutes"=w187:i32)  [unwired: 11 in]
                n85 = Index Array(array=w188, index=w187) -> (element=w186:u16)
                n86 = Quotient & Remainder(x=w186, y=u16 60) -> (x-y*floor(x/y)=→"RunTime_seconds":u16, floor(x/y)=→"RunTime_minutes":u16)
              }
            }
            n87 = case shown="True" w153 {
              tunnel: w152 -> [_ w190]
              tunnel: w151 -> [_ w189]
              frame False {
              }
              frame True {
                n88 = call "myRIO_BRig_Host_parse_dataBlock__v3.vi"("input_dataCurrent"=w189, "input_dataBlock"=w190) -> ("BlockR_T2R_avg"=→"BlockR_T2R_avg":dbl, "BlockR_BTPR_avg"=→"BlockR_BTPR_avg":dbl, "BlockL_BTPR_avg"=→"BlockL_BTPR_avg":dbl, "BlockL_T2R_avg"=→"BlockL_T2R_avg":dbl, "BlockR_BTPR_cur"=→"BlockR_BTPR_cur":u16, "BlockL_BTPR_cur"=→"BlockL_BTPR_cur":u16, "BlockR_T2R_cur"=→"BlockR_T2R_cur":u16, "BlockL_T2R_cur"=→"BlockL_T2R_cur":u16)  [unwired: 2 in]
              }
            }
            n89 = Equal To 0?(x=w126) -> (x = 0?=w125:bool)
            n90 = To Long Integer(number=w120) -> (32bit integer=w119:i32)
            n91 = Select(t=w122, s=w125, f=0) -> (s? t:f=w123:i32)
            n92 = call "myRIO_BRig_Host_comm_getData_2D_u16.vi"("input_fileName"="dataTrial") -> ("output_data_2D"=w145:u16[][], "output_I_data"=w146:bool)  [unwired: 9 in]
            n93 = Increment(x=w119) -> (x+1=w118:i32)
            n94 = case shown="True" w146 {
              tunnel: w145 -> [_ w174]
              tunnel: [w161 w170] -> w141
              tunnel: [w160 w169] -> w140
              tunnel: [w162 w171] -> w142
              tunnel: [w163 w172] -> w143
              tunnel: [w159 w168] -> w139
              tunnel: [w158 w167] -> w138
              tunnel: [w157 w166] -> w137
              tunnel: [w156 w165] -> w136
              tunnel: w127 -> [_ w173]
              tunnel: w135 -> [w163 w182]
              tunnel: w134 -> [w162 w181]
              tunnel: w133 -> [w161 w180]
              tunnel: w132 -> [w160 w179]
              tunnel: w131 -> [w159 w178]
              tunnel: w130 -> [w158 w177]
              tunnel: w129 -> [w157 w176]
              tunnel: w128 -> [w156 w175]
              tunnel: [w155 w164] -> w117
              tunnel: w116 -> [w155 _]
              frame False {
              }
              frame True {
                n95 = call "myRIO_BRig_Host_parse_dataTrial__readMain.vi"("input_idxUnknown"=w182, "input_arrayUnknown"=w181, "input_idxReward"=w180, "input_arrayReward"=w179, "input_idxWrong"=w178, "input_arrayWrong"=w177, "input_idxTimeout"=w176, "input_arrayTimeout"=w175, "arrayIn_dataTrial"=w174, "arrayIn_empty"=w173) -> ("output_countTrial"=w164:i32, "output_idxUnknown"=w172:i32, "output_arrayUnknown"=w171:i32[][], "output_idxReward"=w170:i32, "output_arrayReward"=w169:i32[][], "output_idxWrong"=w168:i32, "output_arrayWrong"=w167:i32[][], "output_idxTimeout"=w166:i32, "output_arrayTimeout"=w165:i32[][])  [unwired: 9 in]
              }
            }
          }
        }
      }
      frame True {
        n96 = Select(t=u32 100 ("milliseconds to wait"), s=w212, f=u32 0 ("milliseconds to wait")) -> (s? t:f=w214:u32)
        n97 = Wait (ms)(milliseconds to wait=w214) -> ()  [unwired: 1 out]
        n98 = case shown="False" w212 {
          tunnel: w211 -> [_ w228]
          frame False {
            n99 = flat-sequence {
              tunnel: ["Select dataExp" ("prompt")] -> w219
              frame #0 {
                n100 = local write "LoadPrevSettings"(FALSE ("LoadPrevSettings")) -> ()
              }
            }
            n101 = call "myRIO_BRig_Host_comm_hostRoot.vi"() -> ("output_hostRoot"=w221:string)  [unwired: 11 in]
            n102 = call "myRIO_BRig_RT_comm_webdav_hostFolder_store.vi"() -> ("output_HostFolder"=w223:string)  [unwired: 11 in]
            n103 = Concatenate Strings(w221, "\\" ("string"), w223) -> (w224:string)
            n104 = String To Path(string=w224) -> (path=w220:path)
            n105 = call "File Dialog"("start path"=w220, "prompt"=w219) -> ("selected path"=w216:path, "exists"=w217:bool, "error out"=→"error_LoadPrevSettings":errorcluster)  [unwired: 10 in, 1 out]
            n106 = case shown="True" w217 {
              tunnel: w216 -> [_ w225]
              frame False {
              }
              frame True {
                n107 = call "myRIO_BRig_Host_comm_webdav_uploadSettings.vi"("input_filePath"=w225) -> ()  [unwired: 11 in]
              }
            }
          }
          frame True {
            n108 = call "myRIO_BRig_Host_endExp_storeFiles__v4_noAnalogLabelling.vi"("input_filePath"=w228) -> ()  [unwired: 15 in]
          }
        }
      }
    }
  }
  n109 = call "myRIO__TCP_disconnect_forRead.vi"("input_error"=w4, "input_hTCP"=w5) -> ("output_error"=→"error_TCP":errorcluster)  [unwired: 9 in]
